vi "Executor.vi"() -> ()   [LabVIEW 2018]
uses:
  QBuilder Files/Actions_arr.ctl
  QBuilder Files/Action.ctl
  QBuilder Files/Parameters.ctl
  Executor Files/MacroInfo.ctl
  Executor Files/Calibrations.ctl
  Executor Files/VariableScan_Cluster.ctl
  Executor Files/RT Actions.ctl
  Executor Files/RT/ActionCluster.ctl
  Executor Files/RT/Instructions_RT.ctl
  Executor Files/RT/ParameterSubCluster.ctl
  Executor Files/State.ctl
  <vilib>/NI/AMC/Message Queue.ctl
  <vilib>/NI/AMC/Message.ctl
  <vilib>/NI/Tools/Keyed Array/KeyedArray.ctl
  Executor Files/RT/Target/Request.ctl
  <vilib>/NI/AMC/Create Single Message.vi
  <vilib>/NI/AMC/Update Message Routing Info.vi
  <vilib>/NI/AMC/Read Termination Message.vi
  <vilib>/NI/AMC/Send Message.vi
  <vilib>/NI/AMC/Globals.vi
  <vilib>/NI/AMC/AMC.lvlib
  <vilib>/NI/Tools/Keyed Array/Tools_KeyedArray.lvlib
panel:
  out "State":T1=enum."idle"
  out "Times (ms)":i64[](array[numeric])
  in  "System":u16(ring)=1 items=["Cusp", "Positron", "Musashi"]
  out "# always zero":i32
  out "error out":errorcluster
  in  "Macro Info 2D":T2(array[cluster])=[[{"Duration (s)"=0.01, "Instruction Description"="Mod 7V", "Input Bits"=[], "Output Bits"=[FALSE, FALSE, FALSE, FALSE, FALSE, FALSE, FALSE, FALSE, FALSE, FALSE, FALSE, FALSE, FALSE, FALSE, FALSE, FALSE, FALSE, FALSE, FALSE, FALSE, FALSE, FALSE, FALSE, FALSE, FALSE, FALSE, FALSE, FALSE, FALSE, FALSE, FALSE, FALSE, FALSE, FALSE, FALSE, FALSE, FALSE, FALSE], "Excitations"=[0.4661287958533758, -0.00044019955713256676, -0.0004811194044810927, -0.0003270089360197006, -0.00037474988790963174, -0.00027444024231065297, -0.0004032935641068728, -0.0003012834675718561, -0.0003574123346967952, -0.0002612820237967628, -0.00044389144836399103, -0.0003012330472735062, -0.00021413562815348174, -0.000348292029470864, -0.0006236629805725628, -0.0003687933751299158, -0.0009869232667160128, -0.00016073401868532967, -0.000402023518375825, -0.0002482954850485854, -0.0003689863609223317, -0.00026807315716459023, -8.725125004194771e-05, -0.00026778601219765283], "Steps"=1, "Changes"=[TRUE, TRUE]}], [{"Duration (s)"=0.1, "Instruction Description"="magnets off (safety)", "Input Bits"=[], "Output Bits"=[FALSE, FALSE, FALSE, FALSE, FALSE, FALSE, FALSE, FALSE, FALSE, FALSE, FALSE, FALSE, FALSE, FALSE, FALSE, FALSE, FALSE, FALSE, FALSE, FALSE, FALSE, FALSE, FALSE, FALSE, FALSE, FALSE, FALSE, FALSE, FALSE, FALSE, FALSE, FALSE, FALSE, FALSE, FALSE, FALSE, FALSE, FALSE], "Excitations"=[0.4661287958533758, -0.00044019955713256676, -0.0004811194044810927, -0.0003270089360197006, -0.00037474988790963174, -0.00027444024231065297, -0.0004032935641068728, -0.0003012834675718561, -0.0003574123346967952, -0.0002612820237967628, -0.00044389144836399103, -0.0003012330472735062, -0.00021413562815348174, -0.000348292029470864, -0.0006236629805725628, -0.0003687933751299158, -0.0009869232667160128, -0.00016073401868532967, -0.000402023518375825, -0.0002482954850485854, -0.0003689863609223317, -0.00026807315716459023, -8.725125004194771e-05, -0.00026778601219765283], "Steps"=1, "Changes"=[TRUE, FALSE]}]] {"Duration (s)" format="%_6p"; "Excitations" format="%_3f"}
  in  "stop":bool
  in  "Tab Control":T3(tab)
  in  "List Cycles":u32
  in  "Cycles":u32
  out "Ping":bool
  out "Sending":bool
  in  "Target stale":bool
  in  "Slave?":bool
  in  "Variable Scan":bool
  in  "Zero All":bool
  out "Time (s)":dbl=5.178 format="%.3f"
  out "% completed":dbl(slide) scale=0.0..1.0
  out "Duration (s)":dbl=0.12200000000000001 format="%.3f"
  in  "Stale":bool
  in  "Run":bool
  out "Cue Description":string="moderator to 7 V"
  in  "Cue Path":path=path "C:/CuspControl/Positron/1_Cues/Util/BiasModerator.q"
  out "Cue Info":T4(array[cluster])=[{"Duration (s)"=0.012, "Action Description"=""}, {"Duration (s)"=0.1, "Action Description"="magnets off (safety)"}] {"Duration (s)" format="%_6p"}
  out "Current\nAction":i32=2
  in  "ABORT":bool
  in  "Favorites":T5(array[cluster])=[{"Cue Path"=path "C:/CuspControl/Positron/1_Cues/RealBaseline/FPS_1s.q", "Slave"=FALSE, "Cycle"=1, "Completed"=0}, {"Cue Path"=path "C:/CuspControl/Positron/1_Cues/RealBaseline/Stack_v23_mcp_1.q", "Slave"=FALSE, "Cycle"=1, "Completed"=0}, {"Cue Path"=path "C:/CuspControl/Positron/1_Cues/Baseline/Stack_v23_s_100.q", "Slave"=FALSE, "Cycle"=1, "Completed"=0}, {"Cue Path"=path "C:/CuspControl/Positron/1_Cues/Util/BiasModerator.q", "Slave"=FALSE, "Cycle"=1, "Completed"=0}]
  out "Timing":i64[](graph)=[18, 2004, 1052, 1052, 1052]
  in  "Skip wait":bool
  in  "Params deadtime (s)":dbl=0.004
  in  "Macro deadtime (s)":dbl=0.006
  out "RepAct#list":i32[](array[numeric])=[0, 1]
  in  "# AO cards":u8=3
  out "# trodes\nin calibr":u8=24
  in  "Save Calibration":bool
  in  "Open Calibration":bool
  in  "Calibrations":T6=[{"Gain"=15.0098, "Offset (V)"=0.0035, "Name"="Vm"}, {"Gain"=14.9932, "Offset (V)"=0.0066, "Name"="in"}, {"Gain"=14.9651, "Offset (V)"=0.0072, "Name"="s1"}, {"Gain"=14.9843, "Offset (V)"=0.0049, "Name"="s2"}, {"Gain"=14.9433, "Offset (V)"=0.0056, "Name"="s3r"}, {"Gain"=14.9395, "Offset (V)"=0.0041, "Name"="s3s"}, {"Gain"=14.8775, "Offset (V)"=0.006, "Name"="s4"}, {"Gain"=14.9361, "Offset (V)"=0.0045, "Name"="g8"}, {"Gain"=15.1086, "Offset (V)"=0.0054, "Name"="e1"}, {"Gain"=14.9264, "Offset (V)"=0.0039, "Name"="c1"}, {"Gain"=14.8685, "Offset (V)"=0.0066, "Name"="c2"}, {"Gain"=14.9386, "Offset (V)"=0.0045, "Name"="c3"}, {"Gain"=14.9438, "Offset (V)"=0.0032, "Name"="c4"}, {"Gain"=14.93, "Offset (V)"=0.0052, "Name"="c5"}, {"Gain"=14.9119, "Offset (V)"=0.0093, "Name"="c6"}, {"Gain"=14.9135, "Offset (V)"=0.0055, "Name"="c7"}, {"Gain"=14.9961, "Offset (V)"=0.0148, "Name"="c8"}, {"Gain"=14.9315, "Offset (V)"=0.0024, "Name"="c9"}, {"Gain"=14.9245, "Offset (V)"=0.006, "Name"="e2"}, {"Gain"=14.9016, "Offset (V)"=0.0037, "Name"="--"}, {"Gain"=14.9057, "Offset (V)"=0.0055, "Name"="--"}, {"Gain"=14.9213, "Offset (V)"=0.004, "Name"="--"}, {"Gain"=14.8995, "Offset (V)"=0.0013, "Name"="--"}, {"Gain"=14.9373, "Offset (V)"=0.004, "Name"="--"}] {"Offset (V)" format="%_6p"; "Gain" format="%_6p"}
  in  "Calibration path":path=path "C:/CuspControl/Positron/Configuration/Calibration/Zz_Gal_to_Area.cal"
  out "# electrodes error":bool=TRUE
  in  "outbits (38)":i32=38
  in  "iswap1_1":i32
  in  "iswap1_2":i32
  in  "iswap2_1":i32
  in  "iswap2_2":i32
  in  "Tab Control 2":T7(tab)=enum."VI Server"
  out "Actions":T8=[{"Toggle"=FALSE, "Open parameter editor"=FALSE, "Open MacroEditor"=FALSE, "Macro path"=path "C:/CuspControl/Positron/1_Macros/Util/Moderator7V.mac", "Duration (s)"=0.012, "Parameters"=[{"Status"="Camera", "Name"="state (0,1)", "Value"=0.0, "Changed"=FALSE}, {"Status"="Slave", "Name"="state (0,1)", "Value"=0.0, "Changed"=FALSE}, {"Status"="Wait", "Name"="inbit (0...7)", "Value"=0.0, "Changed"=FALSE}, {"Status"="Coils", "Name"="buncher (A)", "Value"=0.0, "Changed"=FALSE}, {"Status"="Coils", "Name"="michishio (A)", "Value"=0.0, "Changed"=FALSE}, {"Status"="Coils", "Name"="acorn (A)", "Value"=0.0, "Changed"=FALSE}, {"Status"="Coils", "Name"="stacker (A)", "Value"=0.0, "Changed"=FALSE}, {"Status"="Coils", "Name"="T2 + T3 (A)", "Value"=0.0, "Changed"=FALSE}, {"Status"="Coils", "Name"="T4 (A)  ", "Value"=0.0, "Changed"=FALSE}, {"Status"="Coils", "Name"="-------- (A)", "Value"=0.0, "Changed"=FALSE}, {"Status"="RW", "Name"="mode (0-9)", "Value"=0.0, "Changed"=FALSE}, {"Status"="RW", "Name"="f_start (Hz)", "Value"=0.0, "Changed"=FALSE}, {"Status"="RW", "Name"="f_stop (Hz)", "Value"=0.0, "Changed"=FALSE}, {"Status"="RW", "Name"="amplitude (V)", "Value"=0.0, "Changed"=FALSE}, {"Status"="RW", "Name"="phase dif (deg)", "Value"=0.0, "Changed"=FALSE}, {"Status"="RW", "Name"="sweep time (s)", "Value"=0.0, "Changed"=FALSE}, {"Status"="HVpuls1", "Name"="enable (0,1)", "Value"=0.0, "Changed"=FALSE}, {"Status"="HVpuls1", "Name"="amplitude (V)", "Value"=0.0, "Changed"=FALSE}, {"Status"="HVpuls2", "Name"="enable (0,1)", "Value"=0.0, "Changed"=FALSE}, {"Status"="HVpuls2", "Name"="amplitude (V)", "Value"=0.0, "Changed"=FALSE}, {"Status"="HVpuls3", "Name"="enable (0,1)", "Value"=0.0, "Changed"=FALSE}, {"Status"="HVpuls3", "Name"="amplitude (V)", "Value"=0.0, "Changed"=FALSE}, {"Status"="MCP", "Name"="front bias (V)", "Value"=0.0, "Changed"=FALSE}, {"Status"="MCP", "Name"="back bias (V)", "Value"=0.0, "Changed"=FALSE}, {"Status"="MCP", "Name"="phos bias (V)", "Value"=0.0, "Changed"=FALSE}, {"Status"="posdaq", "Name"="mode (1 or 0)", "Value"=0.0, "Changed"=FALSE}], "Comment"="", "Reps"=1}, {"Toggle"=TRUE, "Open parameter editor"=FALSE, "Open MacroEditor"=FALSE, "Macro path"=path "", "Duration (s)"=0.1, "Parameters"=[{"Status"="Camera", "Name"="state (0,1)", "Value"=0.0, "Changed"=FALSE}, {"Status"="Slave", "Name"="state (0,1)", "Value"=0.0, "Changed"=FALSE}, {"Status"="Wait", "Name"="inbit (0...7)", "Value"=0.0, "Changed"=FALSE}, {"Status"="Coils", "Name"="buncher (A)", "Value"=1e-05, "Changed"=TRUE}, {"Status"="Coils", "Name"="michishio (A)", "Value"=1e-05, "Changed"=TRUE}, {"Status"="Coils", "Name"="acorn (A)", "Value"=1e-05, "Changed"=TRUE}, {"Status"="Coils", "Name"="stacker (A)", "Value"=1e-05, "Changed"=TRUE}, {"Status"="Coils", "Name"="T2 + T3 (A)", "Value"=1e-05, "Changed"=TRUE}, {"Status"="Coils", "Name"="T4 (A)  ", "Value"=1e-05, "Changed"=TRUE}, {"Status"="Coils", "Name"="-------- (A)", "Value"=1e-05, "Changed"=TRUE}, {"Status"="RW", "Name"="mode (0-9)", "Value"=0.0, "Changed"=FALSE}, {"Status"="RW", "Name"="f_start (Hz)", "Value"=0.0, "Changed"=FALSE}, {"Status"="RW", "Name"="f_stop (Hz)", "Value"=0.0, "Changed"=FALSE}, {"Status"="RW", "Name"="amplitude (V)", "Value"=0.0, "Changed"=FALSE}, {"Status"="RW", "Name"="phase dif (deg)", "Value"=0.0, "Changed"=FALSE}, {"Status"="RW", "Name"="sweep time (s)", "Value"=0.0, "Changed"=FALSE}, {"Status"="HVpuls1", "Name"="enable (0,1)", "Value"=0.0, "Changed"=FALSE}, {"Status"="HVpuls1", "Name"="amplitude (V)", "Value"=0.0, "Changed"=FALSE}, {"Status"="HVpuls2", "Name"="enable (0,1)", "Value"=0.0, "Changed"=FALSE}, {"Status"="HVpuls2", "Name"="amplitude (V)", "Value"=0.0, "Changed"=FALSE}, {"Status"="HVpuls3", "Name"="enable (0,1)", "Value"=0.0, "Changed"=FALSE}, {"Status"="HVpuls3", "Name"="amplitude (V)", "Value"=0.0, "Changed"=FALSE}, {"Status"="MCP", "Name"="front bias (V)", "Value"=0.0, "Changed"=FALSE}, {"Status"="MCP", "Name"="back bias (V)", "Value"=0.0, "Changed"=FALSE}, {"Status"="MCP", "Name"="phos bias (V)", "Value"=0.0, "Changed"=FALSE}, {"Status"="posdaq", "Name"="mode (1 or 0)", "Value"=0.0, "Changed"=FALSE}], "Comment"="magnets off (safety)", "Reps"=1}] {"Reps" min=1 step=1; "Parameters"."Value" format="%_6p"; "Duration (s)" min=0.001 step=0.001 format="%_6p"}
  out "Insts per Act":i32[](array[numeric])=[1, 1]
  out "RT Actions":T11=[{"Macro Instructions"=[{"Duration (s)"=0.01, "Steps"=1, "Changes"=[TRUE, TRUE], "Triggers"=[FALSE, FALSE, FALSE, FALSE, FALSE, FALSE, FALSE, FALSE, FALSE, FALSE, FALSE, FALSE, FALSE, FALSE, FALSE, FALSE, FALSE, FALSE, FALSE, FALSE, FALSE, FALSE, FALSE, FALSE, FALSE, FALSE, FALSE, FALSE, FALSE, FALSE, FALSE, FALSE, FALSE, FALSE, FALSE, FALSE, FALSE, FALSE], "RAW cmds 2D"=[[1527, -1, -2, -1, -1, -1, -1, -1], [-1, -1, -1, -1, -1, -1, -2, -1], [-3, -1, -1, -1, -1, -1, 0, -1]]}], "Slow AO Array"=[], "Duration (s)"=0.01, "Toggle"=FALSE}, {"Macro Instructions"=[{"Duration (s)"=0.1, "Steps"=1, "Changes"=[TRUE, FALSE], "Triggers"=[FALSE, FALSE, FALSE, FALSE, FALSE, FALSE, FALSE, FALSE, FALSE, FALSE, FALSE, FALSE, FALSE, FALSE, FALSE, FALSE, FALSE, FALSE, FALSE, FALSE, FALSE, FALSE, FALSE, FALSE, FALSE, FALSE, FALSE, FALSE, FALSE, FALSE, FALSE, FALSE, FALSE, FALSE, FALSE, FALSE, FALSE, FALSE], "RAW cmds 2D"=[[1527, -1, -2, -1, -1, -1, -1, -1], [-1, -1, -1, -1, -1, -1, -2, -1], [-3, -1, -1, -1, -1, -1, 0, -1]]}], "Slow AO Array"=[{"ao line"="ao0", "Duration, Gain, NewVal"=[0.1, 4.0, 0.0, 10.0, 1e-05]}, {"ao line"="ao1", "Duration, Gain, NewVal"=[0.1, 6.0, 0.0, 30.0, 1e-05]}, {"ao line"="ao5", "Duration, Gain, NewVal"=[0.1, 4.0, 0.0, 20.0, 1e-05]}, {"ao line"="ao6", "Duration, Gain, NewVal"=[0.1, 12.0, 0.0, 100.0, 1e-05]}, {"ao line"="ao2", "Duration, Gain, NewVal"=[0.1, 6.0, 0.0, 80.0, 1e-05]}, {"ao line"="ao3", "Duration, Gain, NewVal"=[0.1, 20.0, 0.0, 80.0, 1e-05]}, {"ao line"="ao4", "Duration, Gain, NewVal"=[0.1, 12.0, 0.0, 80.0, 1e-05]}], "Duration (s)"=0.1, "Toggle"=TRUE}] {"Slow AO Array"."Duration, Gain, NewVal" format="%#_3g"}
  in  "Target IP":string="169.254.48.3"
  in  "Target port":u16=6378
  out "AMC error":errorcluster
  in  "Host port":u16=6674
  in  "GUI_AMCname":string="GUI"
  in  "bite size":i32=5000
  in  "milliseconds to wait":u32=2
  out "RT-to-GUI":T15
  out "Scan-to-GUI":T15
  in  "Scan_AMCname":string="SCAN"
  in  "Scan_AMCname":string="LOCAL"
  out "GUI-to-Scan":T15
  out "PXI card names":string[](array[string])=["DIO:", "6509", "Counter:", "6733_1", "Fast AO:", "6733_1", "6733_2", "6733_3", "Slow AO:", "6723"]
  out "DoDogPaths":string[](array[string])=["C:\\CuspControl\\Positron\\DoDogSubVIs\\SourceCoilControl_Wrapper.vi", "C:\\CuspControl\\GPIB and Network\\SourceCoils.txt", "Source Coils enable (1 or 0)", "1", "C:\\CuspControl\\Positron\\DoDogSubVIs\\RGSBias_Wrapper.vi", "C:\\CuspControl\\GPIB and Network\\RGSBias.txt", "Moderator Bias (V)", "1", "C:\\CuspControl\\Positron\\DoDogSubVIs\\HigakiBSetU-I_Wrapper.vi", "C:\\CuspControl\\GPIB and Network\\HigakiB.txt", "Higaki B charge (1 or 0)", "1", "C:\\CuspControl\\Positron\\DoDogSubVIs\\TLSetAllVoltages_Wrapper.vi", "C:\\CuspControl\\GPIB and Network\\TL.txt", "Transfer Line enable (1 or 0)", "1", "C:\\CuspControl\\Positron\\DoDogSubVIs\\TLSetExitCoil_Wrapper.vi", "C:\\CuspControl\\GPIB and Network\\TL.txt", "Only Extr. Coil enable -> on MCP (1 or 0)", "1", "C:\\CuspControl\\Positron\\DoDogSubVIs\\RGSCoilControl_Wrapper.vi", "C:\\CuspControl\\GPIB and Network\\RGSCoils.txt", "RGS Coils enable (1 or 0)", "1", "C:\\CuspControl\\Positron\\DoDogSubVIs\\HVpulser_Wrapper.vi", "C:\\CuspControl\\GPIB and Network\\HVpulser.txt", "Pulser voltage (divided by 160)", "1"]
  in  "Log Files path":path=path "C:/CuspControl/Positron/Log Files"
  in  "Params paths":path[](array[path])=[path "C:/CuspControl/Cusp/Configuration/Parameters.txt", path "C:/CuspControl/Positron/Configuration/Parameters.txt", path "C:/CuspControl/Musashi/Configuration/Parameters.txt"]
  in  "SlaveState Path":path=path "W:/SlaveState.txt"
  out "Active cue path":path=path "C:/CuspControl/Positron/1_Cues/Util/BiasModerator.q"
  out "Txt cmds":string[](array[string])=["Action 0\n", "Action 1\n"]
  out "Macro Info (display)":T16=[{"Duration (s)"=0.01, "Instruction Description"="Mod 7V", "Input Bits"=[], "Output Bits"=[FALSE, FALSE, FALSE, FALSE, FALSE, FALSE, FALSE, FALSE, FALSE, FALSE, FALSE, FALSE, FALSE, FALSE, FALSE, FALSE, FALSE, FALSE, FALSE, FALSE, FALSE, FALSE, FALSE, FALSE, FALSE, FALSE, FALSE, FALSE, FALSE, FALSE, FALSE, FALSE, FALSE, FALSE, FALSE, FALSE, FALSE, FALSE], "Excitations"=[7.0, 0.0, 0.0, 0.0, 0.0, 0.0, 0.0, 0.0, 0.0, 0.0, 0.0, 0.0, 0.0, 0.0, 0.0, 0.0, 1.734723475976807e-18, 0.0, 0.0, 0.0, 0.0, 0.0, 0.0, 0.0], "Steps"=1, "Changes"=[TRUE, TRUE]}] {"Duration (s)" format="%_6p"}
  in  "Variable Cluster":T17={"Values"=[0.10000000000000003, 0.20000000000000004, 0.30000000000000004], "Action"=1, "Inst."=0, "# Elements"=3, "Next Element"=2, "First Val"=0.10000000000000003, "Final Val"=0.30000000000000004, "Update Array"=FALSE, "Description"="", "Variable Type"=0, "Scan Now"=TRUE, "# Act/Inst."=2, "Electrodes_range"=[], "Parameter Name"="RW&f_start (Hz)", "# Passes"=1} {"Variable Type" items=["Duration (s)", "Voltage (V)", "Parameter"]; "Final Val" format="%_6p"; "First Val" format="%_6p"; "Values" format="%_6p"}
  out "Last Modified (when loaded)":timestamp=timestamp(3834924667 s since 1904-01-01)
  # "u13            u12            u11             u10            u9             u8              u7             u6              u5             u4              u3"
  # "swap electrode lines"
  # "swap electrode lines"
  # "0        2       4       6        8      10     12     14"
  # "0        2       4       6        8      10     12     14     16     18      20    22     24     26     28     30     32     34     36"
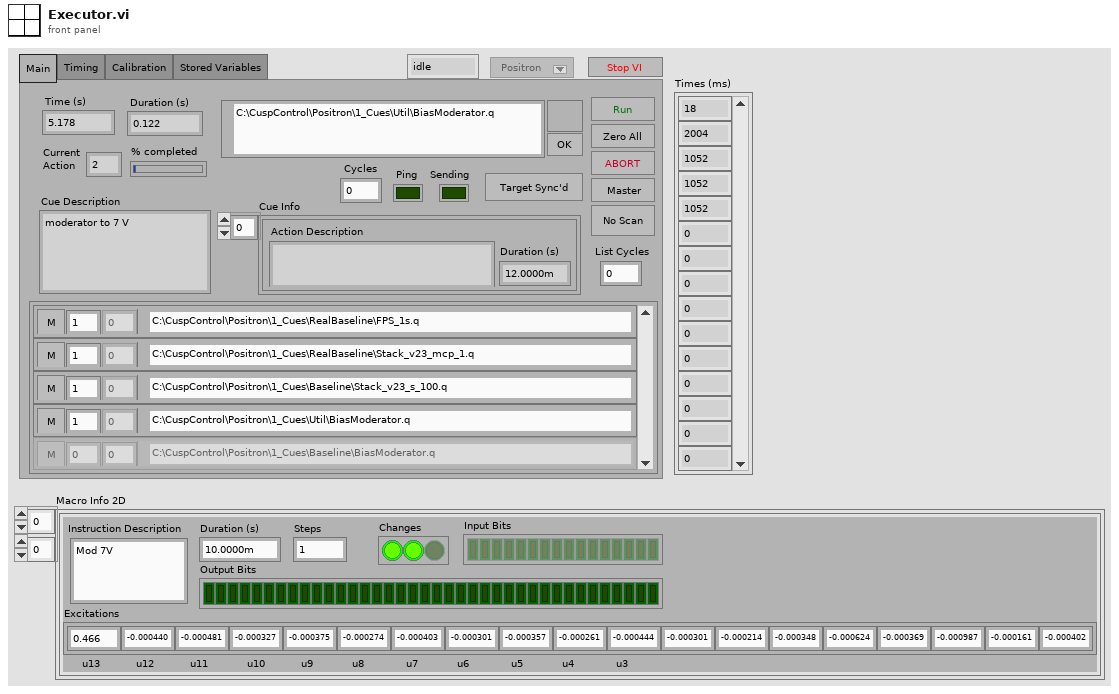
[diagram p1: front panel]
types:
  T1 = typedef "State.ctl" = enum16{"stale", "target stale", "run", "zero all", "open cal", "save cal", "idle"}
  T2 = cluster{"Duration (s)":dbl, "Instruction Description":string, "Input Bits":bool[], "Output Bits":bool[], "Excitations":dbl[], "Steps":i32, "Changes":bool[]}[][]
  T3 = enum32{"Main", "Timing", "Calibration", "Stored Variables"}
  T4 = cluster{"Duration (s)":dbl, "Action Description":string}[]
  T5 = cluster{"Cue Path":path, "Slave":bool, "Cycle":u32, "Completed":u32}[]
  T6 = typedef "Calibrations.ctl" = cluster{"Gain":dbl, "Offset (V)":dbl, "Name":string}[]
  T7 = enum32{"Actions", "RT Actions", "VI Server", "Paths and names", "Text commands", "old display", "variable cluster"}
  T8 = typedef "Actions_arr.ctl" = T9[]
  T9 = typedef "Action.ctl" = cluster{"Toggle":bool, "Open parameter editor":bool, "Open MacroEditor":bool, "Macro path":path, "Duration (s)":dbl, "Parameters":T10, "Comment":string, "Reps":i32}
  T10 = typedef "Parameters.ctl" = cluster{"Status":string, "Name":string, "Value":dbl, "Changed":bool}[]
  T11 = typedef "RT Actions.ctl" = T12[]
  T12 = typedef "ActionCluster.ctl" = cluster{"Macro Instructions":T13, "Slow AO Array":T14, "Duration (s)":dbl, "Toggle":bool}
  T13 = typedef "Instructions_RT.ctl" = cluster{"Duration (s)":dbl, "Steps":i32, "Changes":bool[], "Triggers":bool[], "RAW cmds 2D":i16[][]}[]
  T14 = typedef "ParameterSubCluster.ctl" = cluster{"ao line":string, "Duration, Gain, NewVal":dbl[]}[]
  T15 = typedef "AMC.lvlib/Message Queue.ctl" = refnum<queue>
  T16 = typedef "MacroInfo.ctl" = cluster{"Duration (s)":dbl, "Instruction Description":string, "Input Bits":bool[], "Output Bits":bool[], "Excitations":dbl[], "Steps":i32, "Changes":bool[]}[]
  T17 = typedef "VariableScan_Cluster.ctl" = cluster{"Values":dbl[], "Action":i32, "Inst.":i32, "# Elements":i32, "Next Element":i32, "First Val":dbl, "Final Val":dbl, "Update Array":bool, "Description":string, "Variable Type":u16, "Scan Now":bool, "# Act/Inst.":i32, "Electrodes_range":i32[], "Parameter Name":string, "# Passes":i32}
  T18 = enum32{"Invalid", "Standard", "Closed", "Hidden", "Minimized", "Maximized"}
  T19 = enum8{"Enabled", "Disabled", "Disabled and Grayed Out"}
  T20 = enum16{"open", "replace", "create", "open or create", "replace or create", "replace or create with confirmation"}
  T21 = typedef "Request.ctl" = enum16{"Start", "Run", "Skip Wait", "Pause", "Unpause", "Abort", "Shutdown"}
  T22 = cluster{"Cue Path":path, "Slave":bool, "Cycle":u32, "Completed":u32}
  T23 = cluster{"Total\nTime (s)":dbl, "Cue Description":string}
  T24 = cluster{"Duration (s)":dbl, "Action Description":string}
  T25 = cluster{"Duration (s)":dbl, "Instruction Description":string, "Input Bits":bool[], "Output Bits":bool[], "Excitations":dbl[], "Steps":i32, "Changes":bool[]}
  T26 = typedef "MacroSaveCluster.ctl" = cluster{"Instructions":T27, "Changes":bool[][], "Macro Description":string, "Total Time (s)":dbl, "Samples per sec":dbl}
  T27 = typedef "Instructions.ctl" = T28[]
  T28 = typedef "Instruction.ctl" = cluster{"Duration":dbl, "Comment":string, "Steps":i32, "Edit Potential":bool, "Output Bits":bool[], "Macro Path":path, "Potentials":dbl[], "Inherit?":bool}
  T29 = cluster{"Duration (s)":dbl, "Instruction Description":string, "Input Bits":bool[], "Output Bits":bool[], "Excitations":dbl[], "Steps":i32, "Changes":bool[]}[]
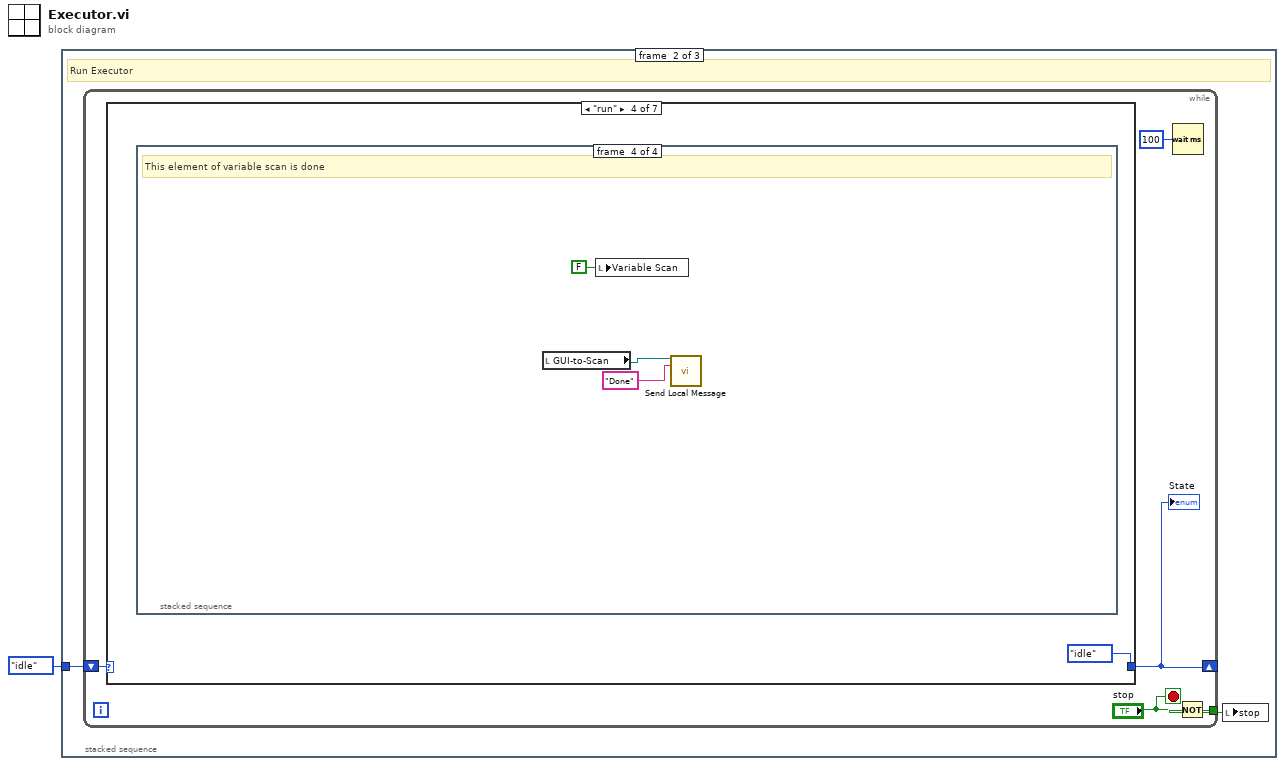
[diagram p0: block diagram]
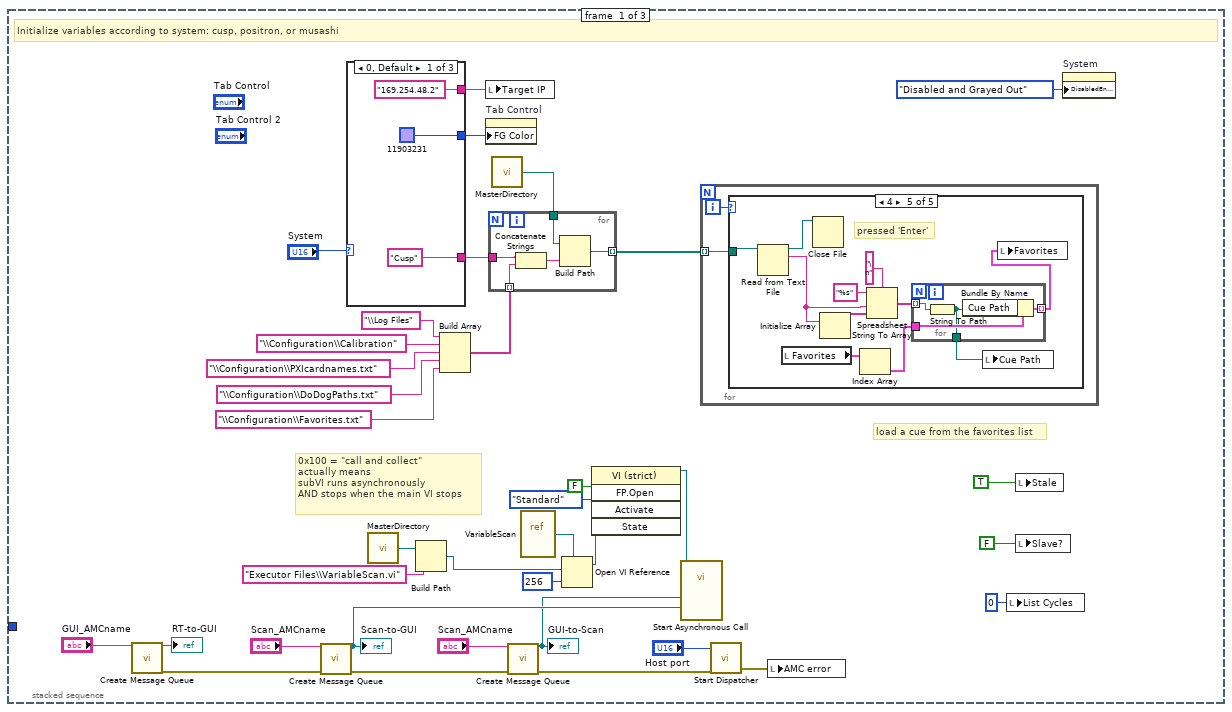
[diagram p2: hidden frame]
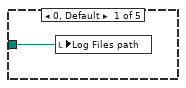
[diagram p3: hidden frame]
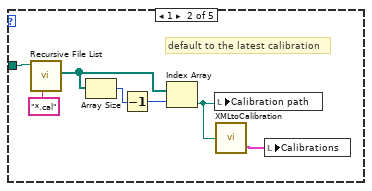
[diagram p4: hidden frame]
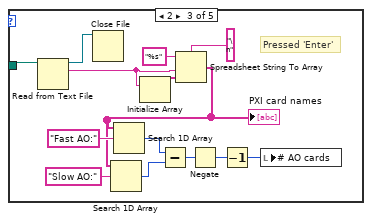
[diagram p5: hidden frame]
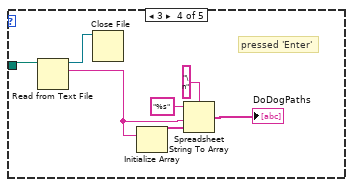
[diagram p6: hidden frame]
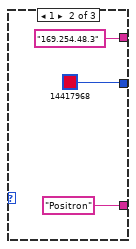
[diagram p7: hidden frame]
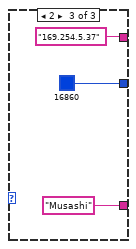
[diagram p8: hidden frame]
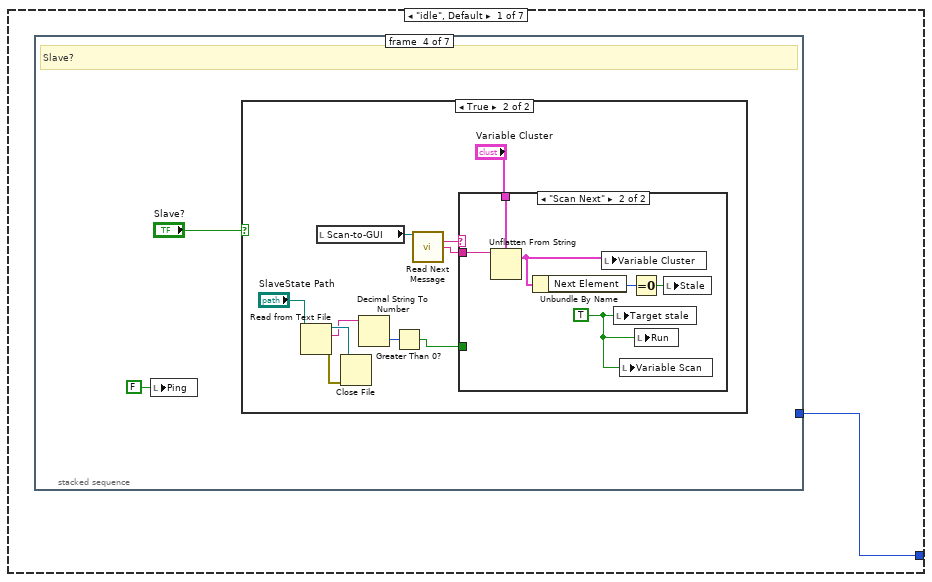
[diagram p9: hidden frame]
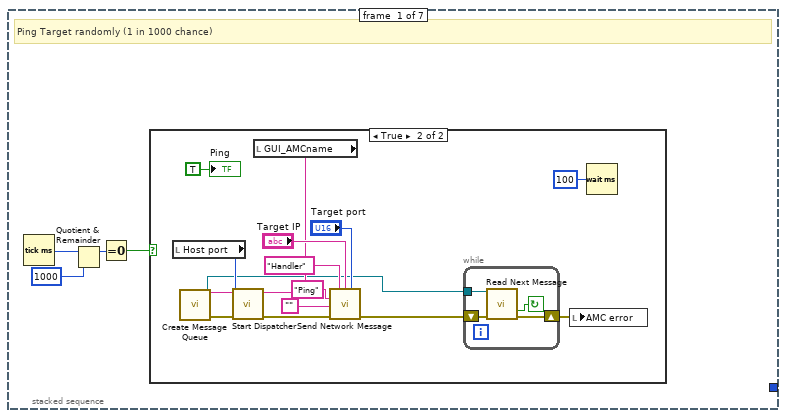
[diagram p10: hidden frame]
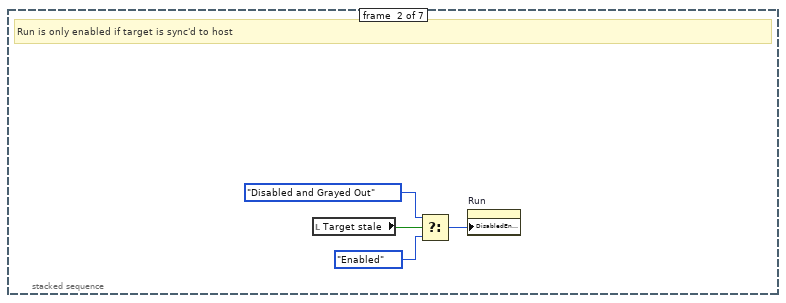
[diagram p12: hidden frame]
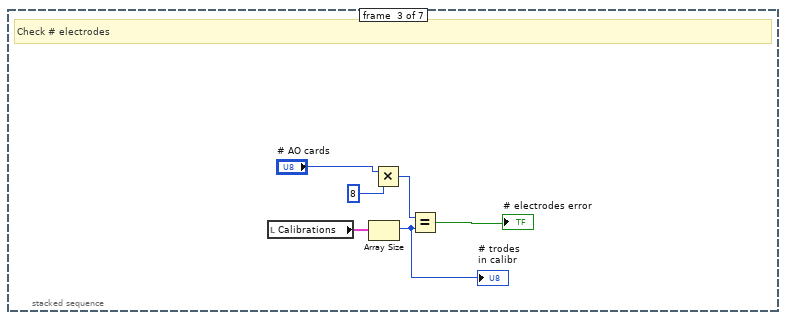
[diagram p13: hidden frame]
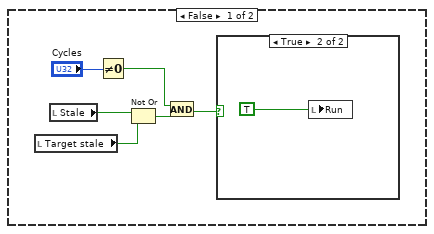
[diagram p14: hidden frame]
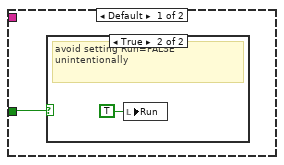
[diagram p16: hidden frame]
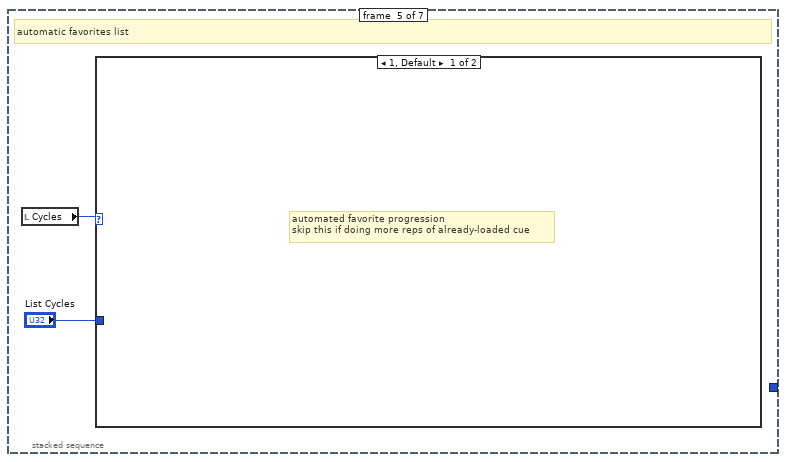
[diagram p18: hidden frame]
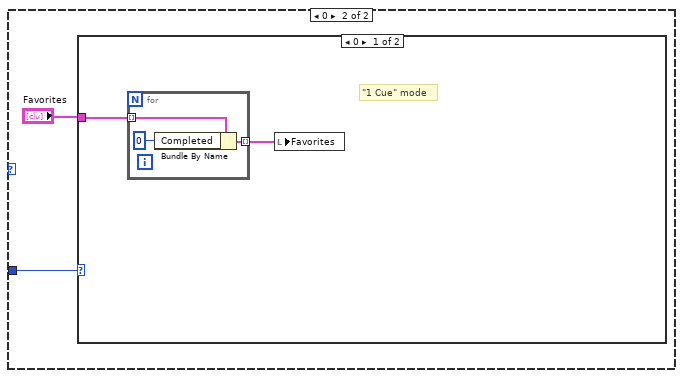
[diagram p19: hidden frame]
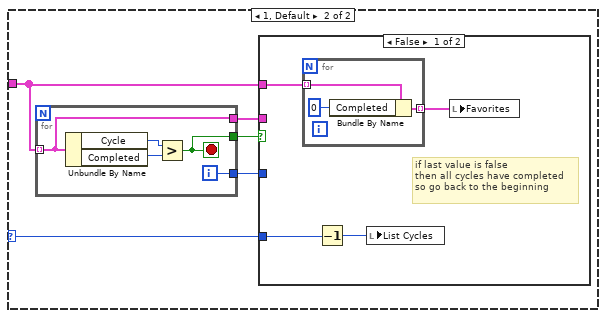
[diagram p20: hidden frame]
diagram:
  n1 = stacked-sequence {
    tunnel: State."idle" ("State") -> [_ w98 _]
    frame #0 {
      # "0x100 = \"call and collect\" \nactually means\nsubVI runs asynchronously\nAND stops when the main VI stops"
      # "load a cue from the favorites list"
      # "Initialize variables according to system: cusp, positron, or musashi"
      n2 = call <vilib>:"Create Message Queue.vi"("message queue name"="GUI_AMCname") -> ("message queue out"=→"RT-to-GUI":T15, "error out"=w17:errorcluster)  [unwired: 13 in]
      n3 = call <vilib>:"Create Message Queue.vi"("message queue name"="Scan_AMCname", "error in"=w17) -> ("message queue out"=w10:T15, "error out"=w13:errorcluster)  [unwired: 12 in]
      "Scan-to-GUI" <- w10
      n4 = case shown="0, Default" "System" {
        tunnel: ["Cusp" ("string") "Positron" ("string") "Musashi" ("string")] -> w33
        tunnel: [u32 11903231 u32 14417968 u32 16860] -> w28
        tunnel: ["169.254.48.2" ("Target IP") "169.254.48.3" ("Target IP") "169.254.5.37" ("Target IP")] -> w27
        frame 0, Default {
        }
        frame 1 {
        }
        frame 2 {
        }
      }
      n5 = call "MasterDirectory.vi"() -> ("Master Directory"=w7:path)
      n6 = Build Path(base path=w7, name or relative path="Executor Files\\VariableScan.vi") -> (appended path=w6:path)
      n7 = Build Array("\\Log Files", "\\Configuration\\Calibration", "\\Configuration\\PXIcardnames.txt", "\\Configuration\\DoDogPaths.txt", "\\Configuration\\Favorites.txt") -> (w32:string[])
      n8 = local write "Target IP"(w27) -> ()
      n9 = property on="Tab Control" class="TabCtl (strict)"("FG Color"=w28) -> ()  [unwired: 2 in, 2 out]
      n10 = call "MasterDirectory.vi"() -> ("Master Directory"=w30:path)
      n11 = for {
        tunnel: w33 -> [w87]
        tunnel: w30 -> [w84]
        tunnel: w32 -> [w86] mode=indexing
        tunnel: [w85] -> w29 mode=indexing
        n12 = Concatenate Strings(w87, w86) -> (w88:string)
        n13 = Build Path(base path=w84, name or relative path=w88) -> (appended path=w85:path)
      }
      n14 = call <vilib>:"Create Message Queue.vi"("message queue name"="Scan_AMCname", "error in"=w13) -> ("message queue out"=w9:T15, "error out"=w16:errorcluster)  [unwired: 12 in]
      "GUI-to-Scan" <- w9
      n15 = vi-ref "VariableScan.vi"() -> (w12:refnum<vi>)
      n16 = Open VI Reference(type specifier VI Refnum (for type only)=w12, vi path=w6, options=256) -> (vi reference=w5:refnum<vi>)  [unwired: 3 in, 1 out]
      n17 = invoke class="VI (strict)" method="FP.Open"(reference=w5, "Activate"=FALSE ("Activate?"), "State"=T18."Standard") -> (reference out=w2:refnum<vi>)  [unwired: 2 in, 4 out]
      n18 = call-by-ref "Start Asynchronous Call"(reference=w2, "Scan-to-GUI"=w10, "GUI-to-Scan"=w9) -> ()  [unwired: 2 in, 2 out]
      n19 = for {
        tunnel: w29 -> [w38] mode=indexing
        i -> [w39]
        n20 = case shown="4" w39 {
          tunnel: w38 -> [w40 w42 w57 w64 w75]
          frame 0, Default {
            n21 = local write "Log Files path"(w40) -> ()
          }
          frame 1 {
            # "default to the latest calibration"
            n22 = call <vilib>:"Recursive File List.vi"("pattern"="*.cal", "Folder Path"=w42) -> ("All Files in Dir"=w41:path[])  [unwired: 5 in, 4 out]
            n23 = Array Size(array=w41) -> (size(s)=w45:i32)
            n24 = Decrement(x=w45) -> (x-1=w44:i32)
            n25 = Index Array(array=w41, index=w44) -> (element=w47:path)
            n26 = local write "Calibration path"(w47) -> ()
            n27 = call "XMLtoCalibration.vi"("XML File Path"=w47) -> ("Calibrations"=w46:T6)  [unwired: 1 in]
            n28 = local write "Calibrations"(w46) -> ()
          }
          frame 2 {
            # "Pressed 'Enter'"
            n29 = Read from Text File(file (use dialog)=w57) -> (refnum out=w61:refnum<file>, text=w59:string)  [unwired: 3 in, 2 out]
            n30 = Close File(refnum=w61) -> ()  [unwired: 1 in, 2 out]
            n31 = Initialize Array(w59) -> (w60:string[])  [unwired: 1 in]
            n32 = Spreadsheet String To Array(delimiter (Tab)="\n", format string="%s", spreadsheet string=w59, array type (2D Dbl)=w60) -> (array=w55:string[])
            "PXI card names" <- w55
            n33 = Search 1D Array(1D array=w55, element="Slow AO:") -> (index of element=w52:i32)  [unwired: 1 in]
            n34 = Search 1D Array(1D array=w55, element="Fast AO:") -> (index of element=w53:i32)  [unwired: 1 in]
            n35 = Subtract(x=w53, y=w52) -> (x-y=w51:i32)
            n36 = Negate(x=w51) -> (-x=w50:i32)
            n37 = Decrement(x=w50) -> (x-1=w49:i32)
            n38 = local write "# AO cards"(w49) -> ()
          }
          frame 3 {
            # "pressed 'Enter'"
            n39 = Read from Text File(file (use dialog)=w64) -> (refnum out=w68:refnum<file>, text=w66:string)  [unwired: 3 in, 2 out]
            n40 = Close File(refnum=w68) -> ()  [unwired: 1 in, 2 out]
            n41 = Initialize Array(w66) -> (w67:string[])  [unwired: 1 in]
            n42 = Spreadsheet String To Array(delimiter (Tab)="\n", format string="%s", spreadsheet string=w66, array type (2D Dbl)=w67) -> (array=→"DoDogPaths":string[])
          }
          frame 4 {
            # "pressed 'Enter'"
            n43 = Read from Text File(file (use dialog)=w75) -> (refnum out=w79:refnum<file>, text=w77:string)  [unwired: 3 in, 2 out]
            n44 = local read "Favorites"() -> (w73:T5)
            n45 = Close File(refnum=w79) -> ()  [unwired: 1 in, 2 out]
            n46 = Initialize Array(w77) -> (w78:string[])  [unwired: 1 in]
            n47 = Index Array(array=w73) -> (element=w72:T22)  [unwired: 1 in]
            n48 = Spreadsheet String To Array(delimiter (Tab)="\n", format string="%s", spreadsheet string=w77, array type (2D Dbl)=w78) -> (array=w71:string[])
            n49 = for {
              tunnel: w72 -> [w83]
              tunnel: w71 -> [w81] mode=indexing
              tunnel: [w82] -> w70 mode=indexing
              tunnel: [w80] -> w69
              n50 = String To Path(string=w81) -> (path=w80:path)
              n51 = Bundle By Name(cluster=w83, "Cue Path"=w80) -> (w82:T22)
            }
            n52 = local write "Cue Path"(w69) -> ()
            n53 = local write "Favorites"(w70) -> ()
          }
        }
      }
      n54 = call <vilib>:"Start Dispatcher.vi"("UDP port (0)"="Host port", "error in"=w16) -> ("error out"=w20:errorcluster)  [unwired: 11 in, 2 out]
      n55 = local write "AMC error"(w20) -> ()
      n56 = local write "List Cycles"(u32 0 ("List Cycles")) -> ()
      n57 = local write "Stale"(TRUE ("Target stale")) -> ()
      n58 = local write "Slave?"(FALSE ("Target stale")) -> ()
      n59 = property on="System" class="Ring (strict)"("DisabledEnum"=T19."Disabled and Grayed Out" ("Disabled")) -> ()  [unwired: 2 in, 2 out]
    }
    frame #1 {
      # "Run Executor"
      n60 = while {
        tunnel: [w104] -> w99
        shift-right: [w101] -> _
        shift-left: w98 -> [w102]
        stop <- "stop" stop-if-true
        n61 = case shown="\"run\"" w102 {
          tunnel: [w105 State."target stale" ("State") w378 State."idle" ("State") State."idle" ("State") State."stale" ("State") State."idle" ("State")] -> w101
          frame "idle", Default {
            n62 = stacked-sequence {
              tunnel: [_ _ _ _ _ _ w225] -> w105
              frame #0 {
                # "Ping Target randomly (1 in 1000 chance)"
                n63 = Tick Count (ms)() -> (millisecond timer value=w109:u32)
                n64 = Quotient & Remainder(x=w109, y=u32 1000) -> (x-y*floor(x/y)=w107:u32)  [unwired: 1 out]
                n65 = Equal To 0?(x=w107) -> (x = 0?=w106:bool)
                n66 = case shown="True" w106 {
                  frame False {
                  }
                  frame True {
                    n67 = local read "Host port"() -> (w114:u16)
                    n68 = local read "GUI_AMCname"() -> (w113:string)
                    n69 = call <vilib>:"Create Message Queue.vi"("message queue name"=w113) -> ("message queue out"=w110:T15, "error out"=w115:errorcluster)  [unwired: 13 in]
                    n70 = call <vilib>:"Start Dispatcher.vi"("UDP port (0)"=w114, "error in"=w115) -> ("error out"=w112:errorcluster)  [unwired: 11 in, 2 out]
                    n71 = call <vilib>:"Send Network Message.vi"("receiver process"="Handler", "receiver host"="Target IP", "receiver port (0)"="Target port", "message name"="Ping" ("String"), "message value"="", "error in"=w112) -> ("error out"=w111:errorcluster)  [unwired: 7 in, 2 out]
                    n72 = while {
                      shift-right: [w126] -> w116
                      shift-left: w111 -> [w127]
                      tunnel: w110 -> [w124]
                      stop <- w125 continue-if-true
                      n73 = call <vilib>:"Read Next Message.vi"("message queue in"=w124, "error in"=w127) -> ("timed out?"=w125:bool, "error out"=w126:errorcluster)  [unwired: 6 in, 6 out]
                    }
                    n74 = local write "AMC error"(w116) -> ()
                    n75 = Wait (ms)(milliseconds to wait=u32 100) -> ()  [unwired: 1 out]
                    "Ping" <- TRUE ("Ping")
                  }
                }
              }
              frame #1 {
                # "Run is only enabled if target is sync'd to host"
                n76 = local read "Target stale"() -> (w128:bool)
                n77 = Select(t=T19."Disabled and Grayed Out" ("Disabled"), s=w128, f=T19."Enabled" ("Disabled")) -> (s? t:f=w131:T19)
                n78 = property on="Run" class="Bool (strict)"("DisabledEnum"=w131) -> ()  [unwired: 2 in, 2 out]
              }
              frame #2 {
                # "Check # electrodes"
                n79 = local read "Calibrations"() -> (w137:T6)
                n80 = Array Size(array=w137) -> (size(s)=w132:i32)
                "# trodes\nin calibr" <- w132
                n81 = Multiply(x="# AO cards", y=u8 8) -> (x*y=w135:u8)
                n82 = Equal?(x=w135, y=w132) -> (x = y?=→"# electrodes error":bool)
              }
              frame #3 {
                # "Slave?"
                n83 = local write "Ping"(FALSE ("Ping")) -> ()
                n84 = case shown="True" "Slave?" {
                  frame False {
                    n85 = local read "Target stale"() -> (w144:bool)
                    n86 = local read "Stale"() -> (w140:bool)
                    n87 = Not Equal To 0?(x="Cycles") -> (x != 0?=w142:bool)
                    n88 = Not Or(1:w144, 2:w140) -> (0:w143:bool)
                    n89 = And(x=w142, y=w143) -> (x .and. y?=w141:bool)
                    n90 = case shown="True" w141 {
                      frame False {
                      }
                      frame True {
                        n91 = local write "Run"(TRUE ("Value (Signaling)")) -> ()
                      }
                    }
                  }
                  frame True {
                    n92 = Read from Text File(file (use dialog)="SlaveState Path") -> (refnum out=w155:refnum<file>, text=w153:string, error out=w154:errorcluster)  [unwired: 3 in, 1 out]
                    n93 = local read "Scan-to-GUI"() -> (w149:T15)
                    n94 = Close File(refnum=w155, error in=w154) -> ()  [unwired: 2 out]
                    n95 = Decimal String To Number(string=w153) -> (number=w152:i32)  [unwired: 2 in, 1 out]
                    n96 = Greater Than 0?(x=w152) -> (x > 0?=w151:bool)
                    n97 = call <vilib>:"Read Next Message.vi"("message queue in"=w149) -> ("message name"=w148:string, "message value"=w147:string)  [unwired: 7 in, 6 out]
                    n98 = case shown="\"Scan Next\"" w148 {
                      tunnel: "Variable Cluster" -> [_ w164]
                      tunnel: w151 -> [w157 _]
                      tunnel: w147 -> [_ w163]
                      frame Default {
                        n99 = case shown="True" w157 {
                          frame False {
                          }
                          frame True {
                            # "avoid setting Run=FALSE \nunintentionally"
                            n100 = local write "Run"(TRUE ("Run")) -> ()
                          }
                        }
                      }
                      frame "Scan Next" {
                        w162 = TRUE ("Value (Signaling)")
                        n101 = Unflatten From String(type=w164, binary string=w163) -> (value=w161:T17)  [unwired: 3 in, 2 out]
                        n102 = Unbundle By Name(w161) -> ("Next Element"=w159:i32)
                        n103 = local write "Variable Cluster"(w161) -> ()
                        n104 = local write "Target stale"(w162) -> ()
                        n105 = local write "Variable Scan"(w162) -> ()
                        n106 = Equal To 0?(x=w159) -> (x = 0?=w160:bool)
                        n107 = local write "Run"(w162) -> ()
                        n108 = local write "Stale"(w160) -> ()
                      }
                    }
                  }
                }
              }
              frame #4 {
                # "automatic favorites list"
                n109 = local read "Cycles"() -> (w166:u32)
                n110 = case shown="1, Default" w166 {
                  tunnel: "List Cycles" -> [_ w168]
                  frame 1, Default {
                    # "automated favorite progression\nskip this if doing more reps of already-loaded cue"
                  }
                  frame 0 {
                    n111 = case shown="0" w168 {
                      selector: w168 -> [_ w174]
                      tunnel: "Favorites" -> [w169 w175]
                      frame 0 {
                        # "\"1 Cue\" mode"
                        n112 = for {
                          tunnel: w169 -> [w172] mode=indexing
                          tunnel: [w171] -> w170 mode=indexing
                          n113 = Bundle By Name(cluster=w172, "Completed"=u32 0) -> (w171:T22)
                        }
                        n114 = local write "Favorites"(w170) -> ()
                      }
                      frame 1, Default {
                        n115 = for {
                          tunnel: w175 -> [w200] mode=indexing
                          tunnel: [w200] -> w178
                          tunnel: [w199] -> w177
                          tunnel: [w196] -> w176
                          i -> [w199]
                          stop <- w196 stop-if-true
                          n116 = Unbundle By Name(w200) -> ("Cycle"=w198:u32, "Completed"=w197:u32)
                          n117 = Greater?(x=w198, y=w197) -> (0:w196:bool)
                        }
                        n118 = case shown="False" w176 {
                          tunnel: w175 -> [w182 w195]
                          tunnel: w178 -> [_ w193]
                          tunnel: w177 -> [_ w194]
                          tunnel: w174 -> [w179 _]
                          frame False {
                            # "if last value is false\nthen all cycles have completed\nso go back to the beginning"
                            n119 = for {
                              tunnel: w182 -> [w184] mode=indexing
                              tunnel: [w183] -> w181 mode=indexing
                              n120 = Bundle By Name(cluster=w184, "Completed"=u32 0) -> (w183:T22)
                            }
                            n121 = Decrement(x=w179) -> (x-1=w180:u32)
                            n122 = local write "List Cycles"(w180) -> ()
                            n123 = local write "Favorites"(w181) -> ()
                          }
                          frame True {
                            n124 = Unbundle By Name(w193) -> ("Cue Path"=w189:path, "Slave"=w188:bool)
                            n125 = Unbundle By Name(w193) -> ("Completed"=w191:u32)
                            n126 = Increment(x=w191) -> (x+1=w190:u32)
                            n127 = local write "Cue Path"(w189) -> ()
                            n128 = local write "Slave?"(w188) -> ()
                            n129 = local write "Cycles"(u32 1 ("Cycles")) -> ()
                            n130 = Bundle By Name(cluster=w193, "Completed"=w190) -> (w192:T22)
                            n131 = Replace Array Subset(array=w195, new element=w192, index=w194) -> (w186:T5)
                            n132 = local write "Favorites"(w186) -> ()
                          }
                        }
                      }
                    }
                  }
                }
              }
              frame #5 {
                # "Check for stale"
                n133 = Empty String/Path?(string/path="Cue Path") -> (empty?=w204:bool)
                n134 = call <vilib>:"Check if File or Folder Exists.vi"("path"="Cue Path") -> ("file or folder exists?"=w202:bool, "dup path"=w206:path)  [unwired: 8 in, 1 out]
                n135 = Not(x=w204) -> (.not. x?=w203:bool)
                n136 = And(x=w202, y=w203) -> (x .and. y?=w201:bool)
                n137 = case shown="True" w201 {
                  tunnel: w206 -> [_ w219]
                  frame False {
                    w207 = u32 0 ("List Cycles")
                    n138 = local read "Favorites"() -> (w212:T5)
                    n139 = Array Size(array=w212) -> (size(s)=w209:i32)
                    n140 = Random Number (0-1)() -> (number: 0 to 1=w211:dbl)
                    n141 = Decrement(x=w209) -> (x-1=w208:i32)
                    n142 = Multiply(x=w208, y=w211) -> (x*y=w214:dbl)
                    n143 = Index Array(array=w212, index=w214) -> (element=w213:T22)
                    n144 = One Button Dialog(message="Invalid path.\nLoading another path from the 'favorites' list") -> ()  [unwired: 1 in, 1 out]
                    n145 = Unbundle By Name(w213) -> ("Cue Path"=w210:path)
                    n146 = local write "List Cycles"(w207) -> ()
                    n147 = local write "Cycles"(w207) -> ()
                    n148 = local write "Cue Path"(w210) -> ()
                  }
                  frame True {
                    n149 = local read "Active cue path"() -> (w220:path)
                    n150 = local read "Last Modified (when loaded)"() -> (w222:timestamp)
                    n151 = File/Directory Info(path=w219) -> (last mod=w221:timestamp, error out=w223:errorcluster)  [unwired: 1 in, 5 out]
                    n152 = Not Equal?(x=w219, y=w220) -> (x != y?=w216:bool)
                    n153 = local write "error out"(w223) -> ()
                    n154 = Not Equal?(x=w222, y=w221) -> (x != y?=w217:bool)
                    n155 = Or(x=w217, y=w216) -> (x .or. y?=w218:bool)
                    n156 = case shown="True" w218 {
                      frame False {
                      }
                      frame True {
                        n157 = local write "Stale"(TRUE ("Stale")) -> ()
                      }
                    }
                  }
                }
              }
              frame #6 {
                # ">> Enum >>"
                # ">> Enum Def >>\n                       V\n                       V"
                # ">> Numeric >>"
                # "update state"
                n158 = Build Array("Stale", "Target stale", "Run", "Zero All", "Open Calibration", "Save Calibration", TRUE ("element")) -> (w232:bool[])
                n159 = for {
                  tunnel: w232 -> [w238] mode=indexing
                  tunnel: [w237] -> w226
                  i -> [w237]
                  stop <- w238 stop-if-true
                }
                n160 = To Variant(anything=w226) -> (Variant=w228:variant)
                n161 = Variant To Data(type=State."stale" ("State"), Variant=w228) -> (data=w225:T1)  [unwired: 1 in, 1 out]
              }
            }
          }
          frame "stale" {
            # "This is the only time that the cue \n(and macros) should be opened from disk"
            n162 = local read "# AO cards"() -> (w246:u8)
            n163 = local write "Stale"(FALSE ("Value (Signaling)")) -> ()
            n164 = Multiply(x=w246, y=u8 8) -> (x*y=w245:u8)
            n165 = Initialize Array(0.0 ("element"), w245) -> (w244:dbl[])
            n166 = Initialize Array(FALSE, "outbits (38)") -> (w247:bool[])
            n167 = stacked-sequence {
              tunnel: w244 -> [_ _ w298 _]
              tunnel: w246 -> [_ _ w297 _]
              tunnel: w247 -> [_ _ w296 _]
              frame #0 {
                # "Update Top Level (Cue)"
                n168 = local read "Cue Path"() -> (w249:path)
                n169 = Empty String/Path?(string/path=w249) -> (empty?=w253:bool)
                n170 = call <vilib>:"Check if File or Folder Exists.vi"("path"=w249) -> ("file or folder exists?"=w250:bool, "dup path"=w255:path)  [unwired: 8 in, 1 out]
                n171 = Not(x=w253) -> (.not. x?=w252:bool)
                n172 = And(x=w250, y=w252) -> (x .and. y?=w251:bool)
                n173 = case shown="False" w251 {
                  tunnel: w255 -> [_ w265]
                  frame False {
                    w256 = u32 0 ("List Cycles")
                    n174 = local read "Favorites"() -> (w262:T5)
                    n175 = Array Size(array=w262) -> (size(s)=w258:i32)
                    n176 = Random Number (0-1)() -> (number: 0 to 1=w261:dbl)
                    n177 = Decrement(x=w258) -> (x-1=w257:i32)
                    n178 = Multiply(x=w257, y=w261) -> (x*y=w264:dbl)
                    n179 = Index Array(array=w262, index=w264) -> (element=w263:T22)
                    n180 = Unbundle By Name(w263) -> ("Cue Path"=w260:path)
                    n181 = local write "List Cycles"(w256) -> ()
                    n182 = local write "Cycles"(w256) -> ()
                    n183 = One Button Dialog(message="Invalid path.\nLoading another path from the 'favorites' list") -> ()  [unwired: 1 in, 1 out]
                    n184 = local write "Cue Path"(w260) -> ()
                  }
                  frame True {
                    n185 = call "XMLtoQ.vi"("XML File Path"=w265) -> ("Cue out"=→"Actions":T8, "Description"=w270:T23)
                    n186 = File/Directory Info(path=w265) -> (last mod=→"Last Modified (when loaded)":timestamp, error out=→"error out":errorcluster)  [unwired: 1 in, 5 out]
                    n187 = Unbundle(w270) -> ("Cue Description"=→"Cue Description":string)  [unwired: 1 out]
                    n188 = local write "Stale"(FALSE ("Stale")) -> ()
                    "Active cue path" <- w265
                  }
                }
                n189 = local write "% completed"(0.0 ("% completed")) -> ()
              }
              frame #1 {
                # "Toggle = TRUE = Change Parameters\nToggle = FALSE = Run a Macro"
                # "Update Mid Level (Actions)"
                n190 = local read "Actions"() -> (w280:T8)
                n191 = local read "Cue Info"() -> (w279:T4)
                n192 = Index Array(array=w279) -> (element=w278:T24)  [unwired: 1 in]
                n193 = for {
                  tunnel: w280 -> [w294] mode=indexing
                  tunnel: [w293] -> w272 mode=indexing
                  tunnel: w278 -> [w292]
                  tunnel: "Macro deadtime (s)" -> [w290]
                  tunnel: "Params deadtime (s)" -> [w289]
                  tunnel: [w284] -> w277 mode=indexing
                  tunnel: [w281] -> w274 mode=concatenating
                  i -> [w283]
                  n194 = Unbundle By Name(w294) -> ("Comment"=w291:string, "Duration (s)"=w288:dbl, "Reps"=w282:i32, "Toggle"=w287:bool)
                  n195 = Bundle By Name(cluster=w292, "Action Description"=w291, "Duration (s)"=w288) -> (w293:T24)
                  n196 = Select(t=w289, s=w287, f=w290) -> (s? t:f=w286:dbl)
                  n197 = Add(x=w288, y=w286) -> (x+y=w285:dbl)
                  n198 = Initialize Array(w283, w282) -> (w281:i32[])
                  n199 = Multiply(x=w282, y=w285) -> (x*y=w284:dbl)
                }
                "RepAct#list" <- w274
                "Cue Info" <- w272
                n200 = Add Array Elements(numeric array=w277) -> (sum=→"Duration (s)":dbl)
              }
              frame #2 {
                # "Update Lower Level (Instructions)"
                n201 = local read "Actions"() -> (w300:T8)
                n202 = local read "Macro Info (display)"() -> (w302:T16)
                n203 = Index Array(array=w302) -> (element=w301:T25)  [unwired: 1 in]
                n204 = for {
                  tunnel: w301 -> [w311]
                  tunnel: [w310] -> w299 mode=indexing
                  tunnel: w300 -> [w309] mode=indexing
                  tunnel: [w308] -> w295 mode=indexing
                  shift-right: [w307] -> _
                  shift-left: w298 -> [w306]
                  tunnel: w297 -> [w305]
                  shift-right: [w304] -> _
                  shift-left: w296 -> [w303]
                  n205 = Unbundle By Name(w309) -> ("Toggle"=w312:bool)
                  n206 = case shown="False" w312 {
                    tunnel: w309 -> [w325 w360]
                    tunnel: [w315 w356] -> w310
                    tunnel: w311 -> [w321 w355]
                    tunnel: [w319 1] -> w308
                    tunnel: [w318 w353] -> w307
                    tunnel: w306 -> [w314 w353]
                    tunnel: w305 -> [w317 _]
                    tunnel: [w316 w352] -> w304
                    tunnel: w303 -> [_ w352]
                    frame False {
                      # "Macro"
                      n207 = Unbundle By Name(w325) -> ("Macro path"=w324:path)
                      n208 = call "XMLtoMacro.vi"("XML File Path"=w324) -> ("MacroSaveCluster"=w323:T26)
                      n209 = Unbundle By Name(w323) -> ("Changes"=w320:bool[][], "Instructions"=w322:T27)
                      n210 = for {
                        tunnel: w322 -> [w348] mode=indexing
                        tunnel: w321 -> [w347]
                        tunnel: [w346] -> w315 mode=indexing
                        tunnel: w320 -> [w330] mode=indexing
                        tunnel: [w342] -> w313
                        tunnel: w317 -> [w341]
                        tunnel: [w340] -> w316
                        shift-right: [w326] -> w318
                        shift-left: w314 -> [w327]
                        n211 = Unbundle By Name(w348) -> ("Duration"=w338:dbl, "Comment"=w339:string, "Output Bits"=w340:bool[], "Steps"=w345:i32, "Potentials"=w343:dbl[])
                        n212 = local read "Calibrations"() -> (w344:T6)
                        n213 = call "ApplyCalibration.vi"("Potentials"=w343, "# AO cards"=w341, "Calibrations"=w344) -> ("# always zero"=w342:i32, "Excitations"=w337:dbl[])  [unwired: 1 in]
                        n214 = call "SwapElectrodes.vi"("index 2"="iswap1_2", "index 1"="iswap1_1", "Excitations in"=w337) -> ("Excitations out"=w334:dbl[])
                        n215 = call "SwapElectrodes.vi"("index 2"="iswap2_2", "index 1"="iswap2_1", "Excitations in"=w334) -> ("Excitations out"=w331:dbl[])
                        n216 = Index Array(array=w330, index=1) -> (element=w328:bool)
                        n217 = Bundle By Name(cluster=w347, "Changes"=w330, "Duration (s)"=w338, "Instruction Description"=w339, "Output Bits"=w340, "Steps"=w345, "Excitations"=w331) -> (w346:T25)
                        n218 = Select(t=w331, s=w328, f=w327) -> (s? t:f=w326:dbl[])
                      }
                      "# always zero" <- w313
                      n219 = Array Size(array=w315) -> (size(s)=w319:i32)
                    }
                    frame True {
                      # "need to carry over excitations\neven for param changes\nbecause ToRAWcmds.vi\ndoesn't discriminate.\n\ndon't need to carry 'changes' or bits\nbecause execution loop does discriminate\n...carry outbits anyway, for display"
                      # "Parameters"
                      n220 = Unbundle By Name(w360) -> ("Duration (s)"=w359:dbl, "Comment"=w358:string)
                      n221 = Initialize Array(FALSE, 0 ("dimension size")) -> (w349:bool[])
                      n222 = Bundle By Name(cluster=w355, "Duration (s)"=w359, "Instruction Description"=w358, "Excitations"=w353, "Input Bits"=w349, "Output Bits"=w352) -> (w357:T25)
                      n223 = Build Array(w357) -> (w356:T29)
                    }
                  }
                }
                "Insts per Act" <- w295
                n224 = local write "Macro Info 2D"(w299) -> ()
              }
              frame #3 {
                # "Update display"
                n225 = local read "Actions"() -> (w365:T8)
                n226 = property on="Cue Info" class="Arr (strict)"() -> ("Index Values"=w364:u32[])  [unwired: 2 in, 2 out]
                n227 = Array Size(array=w365) -> (size(s)=w361:i32)
                n228 = Index Array(array=w364) -> (element=w362:u32)  [unwired: 1 in]
                n229 = Less?(x=w362, y=w361) -> (x < y?=w363:bool)
                n230 = case shown="True" w363 {
                  tunnel: w362 -> [_ w370]
                  frame False {
                  }
                  frame True {
                    n231 = Index Array(array="Macro Info 2D", index (row)=w370) -> (element=w371:T29)  [unwired: 1 in]
                    n232 = local read "# always zero"() -> (w369:i32)
                    n233 = local read "Calibrations"() -> (w368:T6)
                    n234 = for {
                      tunnel: w371 -> [w377] mode=indexing
                      tunnel: [w374] -> w366 mode=indexing
                      tunnel: w369 -> [w373]
                      tunnel: w368 -> [w372]
                      n235 = Unbundle By Name(w377) -> ("Excitations"=w375:dbl[])
                      n236 = call "RemoveCalibration.vi"("Excitations"=w375, "# always zero"=w373, "Calibrations"=w372) -> ("Potentials"=w376:dbl[])  [unwired: 2 in]
                      n237 = Bundle By Name(cluster=w377, "Excitations"=w376) -> (w374:T25)
                    }
                    "Macro Info (display)" <- w366
                  }
                }
              }
            }
          }
          frame "target stale" {
            n238 = local write "Target stale"(FALSE ("Value (Signaling)")) -> ()
            n239 = stacked-sequence {
              seq-local: [_ w400 _ _ _ _] -> [_ _ w411 _ _ _]
              seq-local: [_ w399 _ _ _ _] -> [_ _ w410 _ _ _]
              tunnel: [_ _ _ _ _ w491] -> w378
              frame #0 {
                # "double backslash because \\ is code"
                # "check that the cue matches the system selected on startup"
                n240 = local read "System"() -> (w386:u16)
                n241 = case shown="0, Default" w386 {
                  tunnel: ["CuspControl\\\\Positron" "CuspControl\\\\Musashi" "CuspControl\\\\Cusp"] -> w385
                  frame 1 {
                  }
                  frame 2 {
                  }
                  frame 0, Default {
                  }
                }
                n242 = local read "Cue Path"() -> (w387:path)
                n243 = Path To String(path=w387) -> (string=w384:string)
                n244 = Match Pattern(string=w384, regular expression=w385) -> (offset past match=w383:i32)  [unwired: 1 in, 3 out]
                n245 = Equal?(x=w383, y=-1) -> (x = y?=w381:bool)
                n246 = case shown="True" w381 {
                  tunnel: "Cue must match the system.\nSystem is set at startup, from the dropdown next to Stop VI.\nChange system (Cusp,Positron,Musashi) and start again." ("message") -> [_ w388]
                  frame False {
                  }
                  frame True {
                    n247 = One Button Dialog(message=w388, button name ("OK")="OK") -> (true=w390:bool)
                    n248 = Stop(stop? (T)=w390) -> ()
                  }
                }
              }
              frame #1 {
                # "If Variable Scan, update Actions or Macro Info 2D with new value"
                n249 = local read "Macro Info 2D"() -> (w397:T2)
                n250 = local read "Calibrations"() -> (w395:T6)
                n251 = local read "# always zero"() -> (w396:i32)
                n252 = local read "Actions"() -> (w398:T8)
                n253 = case shown="True" "Variable Scan" {
                  tunnel: [w401 w403] -> w400
                  tunnel: [w402 w404] -> w399
                  tunnel: w398 -> [w402 w407]
                  tunnel: w397 -> [w401 w408]
                  tunnel: w396 -> [_ w406]
                  tunnel: w395 -> [_ w405]
                  frame False {
                  }
                  frame True {
                    n254 = local read "Variable Cluster"() -> (w409:T17)
                    n255 = call "ParamScanSubVI.vi"("Variable Cluster"=w409, "Actions in"=w407, "Macro Info 2D in"=w408, "# always zero"=w406, "Calibrations"=w405) -> ("Actions out"=w404:T8, "Macro Info 2D out"=w403:T2)  [unwired: 5 in]
                    n256 = local write "Macro Info 2D"(w403) -> ()
                    n257 = local write "Actions"(w404) -> ()
                  }
                }
              }
              frame #2 {
                # "Convert all voltage ramps to RAW ramps (interleaved i16's)\nConvert Actions to RT format (Macros only, for now)"
                n258 = local write "Target stale"(TRUE ("Target stale")) -> ()
                n259 = local read "# AO cards"() -> (w416:u8)
                n260 = local read "Insts per Act"() -> (w414:i32[])
                n261 = call "ToRawCommands_RT.vi"("Macro Info 2D"=w411, "# AO cards"=w416) -> ("RAW cluster"=w415:cluster{i16[][]}[][])
                n262 = for {
                  tunnel: w411 -> [w423] mode=indexing
                  tunnel: w415 -> [w422] mode=indexing
                  tunnel: [w417] -> w413 mode=concatenating
                  tunnel: w414 -> [w421] mode=indexing
                  tunnel: w410 -> [w420] mode=indexing
                  n263 = Unbundle By Name(w420) -> ("Toggle"=w419:bool, "Reps"=w418:i32)
                  n264 = for {
                    N: w418 -> [_]
                    tunnel: w423 -> [w429]
                    tunnel: w422 -> [w428]
                    tunnel: w421 -> [w427]
                    tunnel: w419 -> [w425]
                    tunnel: [w424] -> w417 mode=indexing
                    n265 = call "ConvertAction.vi"("RAW cluster 2"=w428, "Macro Info 2D 2"=w429, "Instructions per Action"=w427) -> ("RT Action"=w426:T12)
                    n266 = Bundle(cluster=w426, "Toggle"=w425) -> (w424:T12)  [unwired: 3 in]
                  }
                }
                "RT Actions" <- w413
              }
              frame #3 {
                # "what actually happens in this cue"
                # "list of parameters and their attributes"
                # "start indices of parameter groups"
                # "Write slow AO (target) and txt (local) tables"
                n267 = local read "System"() -> (w446:u16)
                n268 = Index Array(array="Params paths", index=w446) -> (element=w451:path)
                n269 = Read from Text File(file (use dialog)=w451) -> (refnum out=w450:refnum<file>, text=w448:string, error out=w445:errorcluster)  [unwired: 3 in, 1 out]
                n270 = Initialize Array("") -> (w449:string[][])  [unwired: 2 in]
                n271 = Close File(refnum=w450, error in=w445) -> ()  [unwired: 2 out]
                n272 = Spreadsheet String To Array(format string="%s", spreadsheet string=w448, array type (2D Dbl)=w449) -> (array=w440:string[][])  [unwired: 1 in]
                n273 = Index Array(array=w440, index (col)=0 ("disabled index (col)")) -> (element=w444:string[])  [unwired: 1 in]
                n274 = for {
                  tunnel: w444 -> [w455] mode=indexing
                  shift-right: [w455] -> _
                  shift-left: "" -> [w454]
                  tunnel: [w452] -> w443 mode=indexing if=w453
                  tunnel: [w452] -> w435
                  i -> [w452]
                  n275 = Not Equal?(x=w454, y=w455) -> (x != y?=w453:bool)
                }
                n276 = Increment(x=w435) -> (x+1=w434:i32)
                n277 = local read "Actions"() -> (w442:T8)
                n278 = Build Array (concatenate)(w443, w434) -> (w441:i32[])
                n279 = local read "RT Actions"() -> (w437:T11)
                n280 = call "BuildParamSheet.vi"("StartParamIndices"=w441, "Params list"=w440, "Actions"=w442) -> ("DAC cmds"=w438:string[], "txt cmds"=→"Txt cmds":string[])
                n281 = call "AddSlowAO.vi"("RT Actions (without slowAO)"=w437, "DAC cmds"=w438) -> ("RT Actions"=w436:T12[])
                n282 = local write "RT Actions"(w436) -> ()
              }
              frame #4 {
                # "Send cue to RT target in bites that aren't too big for AMC"
                n283 = local read "RT Actions"() -> (w469:T11)
                n284 = Flatten To String(anything=w469) -> (data string=w468:string)  [unwired: 3 in, 2 out]
                n285 = local read "Target IP"() -> (w465:string)
                n286 = call "BreakupString.vi"("bite size"="bite size", "data string"=w468) -> ("Array"=w467:string[])
                n287 = local read "Target port"() -> (w461:u16)
                n288 = disable-structure shown="Enabled" {
                  disable-tunnel: [w471 w476] -> w459
                  disable-tunnel: [w470 errorcluster {"status"=FALSE, "code"=0, "source"=""} ("error out")] -> w457
                  frame Disabled {
                    n289 = local read "GUI_AMCname"() -> (w472:string)
                    n290 = call <vilib>:"Create Message Queue.vi"("message queue name"=w472) -> ("message queue out"=w471:T15, "error out"=w474:errorcluster)  [unwired: 13 in]
                    n291 = local read "Host port"() -> (w473:u16)
                    n292 = call <vilib>:"Start Dispatcher.vi"("UDP port (0)"=w473, "error in"=w474) -> ("error out"=w470:errorcluster)  [unwired: 11 in, 2 out]
                  }
                  frame Enabled {
                    n293 = local read "RT-to-GUI"() -> (w476:T15)
                  }
                }
                n294 = for {
                  tunnel: w461 -> [w490]
                  tunnel: w465 -> [w489]
                  tunnel: "RT Loop" ("receiver process") -> [w487]
                  tunnel: "New Cue" ("String") -> [w486]
                  shift-right: [w484] -> w456
                  shift-left: w457 -> [w488]
                  tunnel: w467 -> [w485] mode=indexing
                  n295 = call <vilib>:"Send Network Message.vi"("receiver process"=w487, "receiver host"=w489, "receiver port (0)"=w490, "message name"=w486, "message value"=w485, "error in"=w488) -> ("error out"=w484:errorcluster)  [unwired: 7 in, 2 out]
                  n296 = Wait (ms)(milliseconds to wait="milliseconds to wait") -> ()  [unwired: 1 out]
                }
                n297 = while {
                  tunnel: w459 -> [w482]
                  shift-right: [w480] -> w458
                  shift-left: w456 -> [w481]
                  stop <- w477 stop-if-true
                  n298 = call <vilib>:"Read Next Message.vi"("message queue in"=w482, "error in"=w481) -> ("message value"=w479:string, "error out"=w480:errorcluster)  [unwired: 6 in, 6 out]
                  n299 = Equal?(x="", y=w479) -> (x = y?=w477:bool)
                }
                n300 = local write "AMC error"(w458) -> ()
                n301 = Wait (ms)(milliseconds to wait=u32 500) -> ()  [unwired: 1 out]
                "Sending" <- TRUE ("Sending")
              }
              frame #5 {
                w493 = FALSE ("Target stale")
                # "autorun if var-scan"
                n302 = local read "Variable Scan"() -> (w492:bool)
                n303 = case shown="True" w492 {
                  tunnel: [State."idle" ("State") State."run" ("State")] -> w491
                  frame False {
                  }
                  frame True {
                  }
                }
                n304 = local write "Target stale"(w493) -> ()
                n305 = local write "Sending"(w493) -> ()
              }
            }
          }
          frame "run" {
            n306 = stacked-sequence {
              frame #0 {
                # "Write to log file; disable Run button until end of Cue"
                n307 = local read "Variable Cluster"() -> (w541:T17)
                n308 = local read "Cue Path"() -> (w537:path)
                n309 = Get Date/Time In Seconds() -> (seconds since 1Jan1904=w527:timestamp)
                n310 = Path To String(path=w537) -> (string=w534:string)
                n311 = Format Date/Time String(time format string (%c)="%H%M%S\\t", seconds (now)=w527) -> (date/time string=w523:string)  [unwired: 1 in]
                n312 = Unbundle By Name(w541) -> ("Variable Type"=w538:u16, "Values"=w540:dbl[], "Next Element"=w531:i32)  [unwired: 3 out]
                n313 = property on="Variable Type" class="Ring (strict)"() -> ("Strings []"=w539:string[])  [unwired: 2 in, 2 out]
                n314 = local read "Variable Scan"() -> (w533:bool)
                n315 = Concatenate Strings(w523, "Cue Path: %s" ("format string")) -> (w524:string)
                n316 = Index Array(array=w539, index=w538) -> (element=w536:string)
                n317 = Index Array(array=w540, index=w531) -> (element=w535:dbl)
                n318 = Concatenate Strings(w524, "\\tParameter: %s\\tValue: %e" ("format string")) -> (w532:string)
                n319 = Get Date/Time In Seconds() -> (seconds since 1Jan1904=w522:timestamp)
                n320 = case shown="True" w533 {
                  tunnel: w536 -> [_ w548]
                  tunnel: w535 -> [_ w547]
                  tunnel: w534 -> [w545 w551]
                  tunnel: [w546 w550] -> w529
                  tunnel: w532 -> [_ w549]
                  tunnel: w524 -> [w544 _]
                  frame False {
                    n321 = Format Into String(format string=w544, w545) -> (resulting string=w546:string)  [unwired: 2 in, 1 out]
                  }
                  frame True {
                    n322 = Format Into String(format string=w549, w551, w548, w547) -> (resulting string=w550:string)  [unwired: 2 in, 1 out]
                  }
                }
                n323 = Format Date/Time String(time format string (%c)="\\%Y-%m-%d.log", seconds (now)=w522) -> (date/time string=w520:string)  [unwired: 1 in]
                n324 = Path To String(path="Log Files path") -> (string=w521:string)
                n325 = Concatenate Strings(w521, w520) -> (w517:string)
                n326 = Concatenate Strings(w529, "\r\n") -> (w502:string)
                n327 = String To Path(string=w517) -> (path=w519:path)
                n328 = call <vilib>:"Check if File or Folder Exists.vi"("path"=w519) -> ("file or folder exists?"=w513:bool, "dup path"=w518:path)  [unwired: 8 in, 1 out]
                n329 = local read "Cycles"() -> (w499:u32)
                n330 = Select(t=T20."open" ("operation (0:open)"), s=w513, f=T20."create" ("operation (0:open)")) -> (s? t:f=w514:T20)
                n331 = property on="ABORT" class="Bool (strict)"("DisabledEnum"=T19."Enabled" ("Disabled")) -> ()  [unwired: 2 in, 2 out]
                n332 = Open/Create/Replace File(file path (use dialog)=w518, operation (0:open)=w514) -> (refnum out=w510:refnum<file>, error out=w509:errorcluster)  [unwired: 4 in, 1 out]
                n333 = Greater Than 0?(x=w499) -> (x > 0?=w500:bool)
                n334 = Read from Text File(file (use dialog)=w510, error in=w509) -> (refnum out=w512:refnum<file>, error out=w511:errorcluster)  [unwired: 2 in, 2 out]
                n335 = case shown="True" w500 {
                  tunnel: w499 -> [_ w542]
                  frame False {
                  }
                  frame True {
                    n336 = Decrement(x=w542) -> (x-1=w543:u32)
                    n337 = local write "Cycles"(w543) -> ()
                  }
                }
                n338 = Set File Position(refnum=w512, from (0:start)=enum16{"start", "end", "current"}."end", error in=w511) -> (refnum out=w508:refnum<file>, error out=w507:errorcluster)  [unwired: 1 in]
                n339 = Write to Text File(file (use dialog)=w508, text=w502, error in=w507) -> (refnum out=w515:refnum<file>, error out=w516:errorcluster)  [unwired: 1 in, 1 out]
                n340 = property on="Run" class="Bool (strict)"("DisabledEnum"=T19."Disabled" ("Disabled")) -> ()  [unwired: 2 in, 2 out]
                n341 = Close File(refnum=w515, error in=w516) -> ()  [unwired: 2 out]
              }
              frame #1 {
                # "Tell Target to run"
                n342 = disable-structure shown="Enabled" {
                  disable-tunnel: [w563 errorcluster {"status"=FALSE, "code"=0, "source"=""} ("error in")] -> w552
                  frame Enabled {
                    n343 = local read "GUI_AMCname"() -> (w562:string)
                    n344 = call <vilib>:"Create Message Queue.vi"("message queue name"=w562) -> ("error out"=w564:errorcluster)  [unwired: 13 in, 1 out]
                    n345 = local read "Host port"() -> (w561:u16)
                    n346 = call <vilib>:"Start Dispatcher.vi"("UDP port (0)"=w561, "error in"=w564) -> ("error out"=w563:errorcluster)  [unwired: 11 in, 2 out]
                  }
                  frame Disabled {
                  }
                }
                n347 = local read "Target port"() -> (w559:u16)
                n348 = local read "Target IP"() -> (w558:string)
                n349 = Flatten To String(anything=Request."Start" ("RT_State")) -> (data string=w554:string)  [unwired: 3 in, 2 out]
                n350 = call <vilib>:"Send Network Message.vi"("receiver process"="RT Loop", "receiver host"=w558, "receiver port (0)"=w559, "message name"="Run Control" ("String"), "message value"=w554, "error in"=w552) -> ("error out"=→"AMC error":errorcluster)  [unwired: 7 in, 2 out]
                n351 = Wait (ms)(milliseconds to wait=u32 100) -> ()  [unwired: 1 out]
              }
              frame #2 {
                w571 = 10000  # Max # of Actions
                # "Follow along with RT execution via AMC\nWrite text files when appropriate Action #'s are reached\nSend commands for interrupting or bypassing part of the Cue"
                n352 = local read "RepAct#list"() -> (w567:i32[])
                n353 = local read "Duration (s)"() -> (w575:dbl)
                n354 = local read "AMC error"() -> (w568:errorcluster)
                n355 = local read "Target port"() -> (w578:u16)
                n356 = local read "RT Actions"() -> (w579:T11)
                n357 = local read "RT-to-GUI"() -> (w566:T15)
                n358 = local read "Target IP"() -> (w577:string)
                n359 = local read "Txt cmds"() -> (w576:string[])
                n360 = Initialize Array(i64 0, w571) -> (w570:i64[])
                n361 = while {
                  tunnel: w579 -> [w599]
                  shift-right: [w596] -> w574
                  shift-left: w568 -> [w604]
                  tunnel: w566 -> [w607]
                  tunnel: w578 -> [w606]
                  tunnel: w577 -> [w605]
                  shift-right: [w601] -> w569
                  shift-left: -1 ("Action # out") -> [w603]
                  tunnel: w576 -> [w600]
                  tunnel: w575 -> [w595]
                  shift-right: [w592] -> _
                  shift-left: w570 -> [w593]
                  tunnel: w567 -> [w591]
                  stop <- w598 stop-if-true
                  n362 = Or(x="ABORT", y="Skip wait") -> (x .or. y?=w589:bool)
                  n363 = call "Comm.vi"("GUI Queue"=w607, "Target port"=w606, "Target IP"=w605, "Action # in"=w603, "Times in"=w593, "error in (no error)"=w604, "Skip wait"=w589) -> ("Next Action?"=w602:bool, "Action # out"=w601:i32, "Times out"=w592:i64[], "error out"=w597:errorcluster)  [unwired: 5 in]
                  n364 = Wait Until Next ms Multiple(millisecond multiple=u32 2) -> ()  [unwired: 1 out]
                  n365 = case shown="False" "Skip wait" {
                    frame False {
                    }
                    frame True {
                      n366 = local write "Skip wait"(FALSE ("Skip wait")) -> ()
                    }
                  }
                  n367 = case shown="False" w602 {
                    tunnel: w601 -> [w612 w621]
                    tunnel: w600 -> [_ w627]
                    tunnel: w599 -> [w614 w626]
                    tunnel: [w616 FALSE] -> w598
                    tunnel: w597 -> [w615 w629]
                    tunnel: [w615 w628] -> w596
                    tunnel: w595 -> [_ w625]
                    tunnel: w592 -> [_ w624]
                    tunnel: "ABORT" -> [w610 _]
                    tunnel: w591 -> [_ w620]
                    frame False {
                      # "continue until last action+1\nto get time of last action"
                      # "if no new action, check for end"
                      n368 = Array Size(array=w614) -> (size(s)=w613:i32)
                      n369 = Less Or Equal?(x=w613, y=w612) -> (x <= y?=w611:bool)
                      n370 = Or(x=w611, y=w610) -> (x .or. y?=w616:bool)
                    }
                    frame True {
                      w622 = i64 1000  # ms per s
                      n371 = call "WriteTextFiles.vi"("error in"=w629, "Action #"=w621, "RT Actions"=w626, "Txt cmds"=w627) -> ("error out"=w628:errorcluster)
                      n372 = Add Array Elements(numeric array=w624) -> (sum=w623:i64)
                      n373 = Index Array(array=w620, index=w621) -> (element=→"Current\nAction":i32)
                      n374 = Divide(x=w623, y=w622) -> (x/y=w619:dbl)
                      "Time (s)" <- w619
                      n375 = Divide(x=w619, y=w625) -> (x/y=→"% completed":dbl)
                      "Times (ms)" <- w624
                      "Timing" <- w624
                    }
                  }
                  n376 = case shown="False" "ABORT" {
                    selector: "ABORT" -> [_ w609]
                    frame False {
                    }
                    frame True {
                      n377 = local write "Zero All"(w609) -> ()
                    }
                  }
                }
                n378 = flat-sequence {
                  tunnel: w574 -> [w582]
                  tunnel: w569 -> [w586]
                  frame #0 {
                    n379 = local read "Timing"() -> (w587:i64[])
                    n380 = local write "AMC error"(w582) -> ()
                    n381 = local write "% completed"(1.0 ("% completed")) -> ()
                    n382 = Array Subset(array=w587, length=w586) -> (w585:i64[])  [unwired: 1 in]
                    n383 = local write "Run"(FALSE ("Execute")) -> ()
                    n384 = property on="Run" class="Bool (strict)"("DisabledEnum"=T19."Enabled" ("Disabled")) -> ()  [unwired: 2 in, 2 out]
                    n385 = property on="ABORT" class="Bool (strict)"("DisabledEnum"=T19."Disabled" ("Disabled")) -> ()  [unwired: 2 in, 2 out]
                    n386 = local write "Timing"(w585) -> ()
                  }
                }
              }
              frame #3 {
                # "This element of variable scan is done"
                n387 = local read "GUI-to-Scan"() -> (w632:T15)
                n388 = local write "Variable Scan"(FALSE ("Variable Scan")) -> ()
                n389 = call <vilib>:"Send Local Message.vi"("message queue in"=w632, "message name"="Done" ("Message Name")) -> ()  [unwired: 11 in, 3 out]
              }
            }
          }
          frame "zero all" {
            # "this command is sent directly to RT Loop\nwhen received, a 0 V cue replaces the cue previously in memory on target\ntarget proceeds to run that as soon as it finishes the last Action"
            n390 = flat-sequence {
              frame #0 {
                n391 = local read "error out"() -> (w636:errorcluster)
                n392 = local read "Target IP"() -> (w641:string)
                n393 = local read "Target port"() -> (w640:u16)
                n394 = call <vilib>:"Send Network Message.vi"("receiver process"="RT Loop", "receiver host"=w641, "receiver port (0)"=w640, "message name"="Zero All", "error in"=w636) -> ("error out"=w635:errorcluster)  [unwired: 8 in, 2 out]
                n395 = local write "error out"(w635) -> ()
                n396 = Wait (ms)(milliseconds to wait=u32 300) -> ()  [unwired: 1 out]
              }
              frame #1 {
                w643 = FALSE
                n397 = local write "Zero All"(w643) -> ()
                n398 = local write "Stale"(TRUE ("Target stale")) -> ()
                n399 = local write "ABORT"(w643) -> ()
                n400 = local write "Run"(w643) -> ()
              }
            }
          }
          frame "open cal" {
            n401 = flat-sequence {
              frame #0 {
                # "wait so that user\nsees that button was\npressed"
                n402 = Wait (ms)(milliseconds to wait=u32 100) -> ()  [unwired: 1 out]
              }
              frame #1 {
                n403 = local write "Open Calibration"(FALSE ("Save Calibration")) -> ()
                n404 = call "XMLtoCalibration.vi"("XML File Path"="Calibration path") -> ("Calibrations"=w649:T6)  [unwired: 1 in]
                n405 = local write "Stale"(TRUE ("Save Calibration")) -> ()
                n406 = local write "Calibrations"(w649) -> ()
              }
            }
          }
          frame "save cal" {
            n407 = local read "Calibration path"() -> (w653:path)
            n408 = local write "Save Calibration"(FALSE ("Save Calibration")) -> ()
            n409 = call "CalibrationtoXML.vi"("Calibrations"="Calibrations", "XML File Path"=w653) -> ()  [unwired: 1 out]
          }
        }
        "State" <- w101
        n410 = Wait (ms)(milliseconds to wait=u32 100) -> ()  [unwired: 1 out]
        n411 = Not(x="stop") -> (.not. x?=w104:bool)
      }
      n412 = local write "stop"(w99) -> ()
    }
    frame #2 {
      # "cleanup"
      n413 = local read "AMC error"() -> (w654:errorcluster)
      n414 = call <vilib>:"Stop Dispatcher.vi"("error in"=w654) -> ("error out"=w655:errorcluster)  [unwired: 14 in]
      n415 = property on="System" class="Ring (strict)"("DisabledEnum"=T19."Enabled" ("Disabled")) -> ()  [unwired: 2 in, 2 out]
      n416 = local write "AMC error"(w655) -> ()
    }
  }
